vi "PH_HamamatsuCamera.set Config.vi"(0 "VI in":refnum<vi>, 1 "Cam Handle in":i32, 4 "Cam Error in":errorcluster, 5 "error in":errorcluster) -> (14 "VI out":refnum<vi>, 15 "Cam Handle out":i32, 18 "Cam Error out":errorcluster, 19 "error out":errorcluster)   [LabVIEW 2014, in "PH_HamamatsuCamera.lvlib"]
uses:
  PH_HamamatsuCamera.lvlib
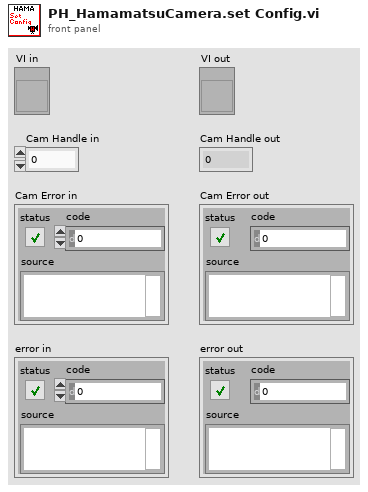
[diagram p1: front panel]
types:
  T1 = typedef "PH_HamamatsuCamera.lvlib/PH_HamamatsuCamera.i attribute.ctl" = cluster{"Gui Refs":cluster{"Camera Details":refnum<vi>, "ROI":refnum<vi>, "Set ROI to Maximum":refnum<vi>, "Trigger Parameters":refnum<vi>, "Brightness":refnum<vi>, "Shutter":refnum<vi>, "Gain":refnum<vi>, "Trigger Timeout":refnum<vi>, "Trigger Polarity":refnum<vi>, "Trigger Mode":refnum<vi>, "Parameters":refnum<vi>, "Set Cam Parameter":refnum<vi>, "Parameter to set":refnum<vi>, "Value to set":refnum<vi>}, "Cam":cluster{"Handle":i32, "Details":cluster{"Model":string, "Camera ID":string, "Firmware":string}, "Buffer Info":cluster{"height":u32, "width":u32, "datatype":u32}}, "H Offset":cluster{"Value":i32, "Minimum":i32, "Maximum":i32, "Increment":i32}, "V Offset":cluster{"Value":i32, "Minimum":i32, "Maximum":i32, "Increment":i32}, "H Width":cluster{"Value":i32, "Minimum":i32, "Maximum":i32, "Increment":i32}, "V Width":cluster{"Value":i32, "Minimum":i32, "Maximum":i32, "Increment":i32}, "Trigger Parameters":T2, "Trigger Timeout":u32, "Parameters":T3[], "Indicees Cam Parameters":cluster{"Brightness":i32, "Shutter":i32, "Gain":i32}, "Wanted Values":cluster{"Trigger Settings":T2[], "ROI":T4[], "Parameter":cluster{"Name":string, "Value":dbl}[]}}
  T2 = typedef "PH_HamamatsuCamera.lvlib/PH_HamamatsuCamera.Trigger Parameter.ctl" = cluster{"Mode":u32, "Polarity":u32, "Times":u32, "Delay":dbl}
  T3 = typedef "PH_HamamatsuCamera.lvlib/PH_HamamatsuCamera.Parameter Set.ctl" = cluster{"Parameter":string, "Value":dbl, "Writable":bool, "Range":cluster{"min":dbl, "max":dbl, "step":dbl}, "Default":dbl, "Value Names":cluster{"Name":string, "Value":dbl}[], "Text Values":bool}
  T4 = typedef "PH_HamamatsuCamera.lvlib/PH_HamamatsuCamera.ROI.ctl" = cluster{"Horizontal Offset":i32, "Vertical Offset":i32, "Horizontal Width":i32, "Vertical Width":i32}
  T5 = cluster{"height":u32, "width":u32, "datatype":u32}
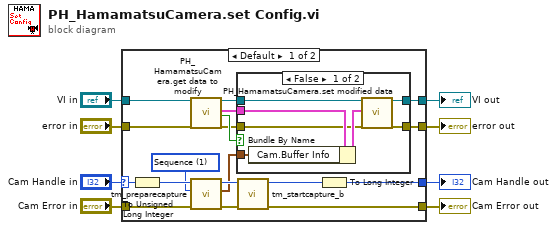
[diagram p0: block diagram]
diagram:
  n1 = case shown="Default" "Cam Handle in" {
    selector: "Cam Handle in" -> [w25 w36]
    tunnel: "VI in" -> [w15 w39]
    tunnel: "error in" -> [w16 w38]
    tunnel: [w14 w39] -> w6
    tunnel: [w13 w38] -> w5
    tunnel: [w12 w37] -> w4
    tunnel: [w9 w36] -> w7
    tunnel: "Cam Error in" -> [w10 w37]
    frame Default {
      w22 = 1 items=["Snap", "Sequence"] ("Capture mode")
      n2 = To Unsigned Long Integer(number=w25) -> (unsigned 32bit integer=w24:u32)
      n3 = call "PH_HamamatsuCamera.get data to modify.vi"("i ref in"=w15, "error in (no error)"=w16) -> ("i ref out"=w21:refnum<vi>, "i attribute"=w20:T1, "timed out"=w19:bool, "error out"=w18:errorcluster)  [unwired: 14 in]
      n4 = call <userlib>:"tm_preparecapture.vi"("error in (no error)"=w10, "Capture mode"=w22, "Handle in"=w24) -> ("error out"=w26:errorcluster, "Buffer Info"=w17:T5, "Handle out"=w23:u32)  [unwired: 5 in, 1 out]
      n5 = case shown="False" w19 {
        tunnel: w18 -> [w27 w34]
        tunnel: w21 -> [w33 w35]
        tunnel: [w32 w35] -> w14
        tunnel: [w31 w34] -> w13
        tunnel: w20 -> [w28 _]
        tunnel: w17 -> [w29 _]
        frame False {
          n6 = Bundle By Name(cluster=w28, "Cam.Buffer Info"=w29) -> (w30:T1)
          n7 = call "PH_HamamatsuCamera.set modified data.vi"("i ref in"=w33, "i attribute"=w30, "error in (no error)"=w27) -> ("i ref out"=w32:refnum<vi>, "error out"=w31:errorcluster)  [unwired: 15 in]
        }
        frame True {
        }
      }
      n8 = call <userlib>:"tm_startcapture_b.vi"("error in (no error)"=w26, "Handle in"=w23) -> ("error out"=w12:errorcluster, "Handle out"=w11:u32)  [unwired: 8 in]
      n9 = To Long Integer(number=w11) -> (32bit integer=w9:i32)
    }
    frame -1 {
    }
  }
  "Cam Handle out" <- w7
  "VI out" <- w6
  "error out" <- w5
  "Cam Error out" <- w4
